vi "Do.vi"(8 "error in (no error)":errorcluster, 10 "Actor in":refnum<class "Actor.lvclass">, 11 "lfieldpanel_acquire_single_frame Msg":refnum<class "lfieldpanel_acquire_single_frame Msg.lvclass">) -> (0 "error out":errorcluster, 2 "Actor out":refnum<class "Actor.lvclass">)   [LabVIEW 2015, in "lfieldpanel_acquire_single_frame Msg.lvclass"]
doc: "This VI delivers the message to the actor by calling the appropriate method(s) on the actor."
uses:
  lfieldpanel_acquire_single_frame Msg.lvclass
  <vilib>/ActorFramework/Actor/Actor.lvclass
  lightfield_panel/lightfield_panel.lvclass
  lfieldpanel_acquire_single_frame Msg.lvclass/lfieldpanel_acquire_single_frame Msg.ctl
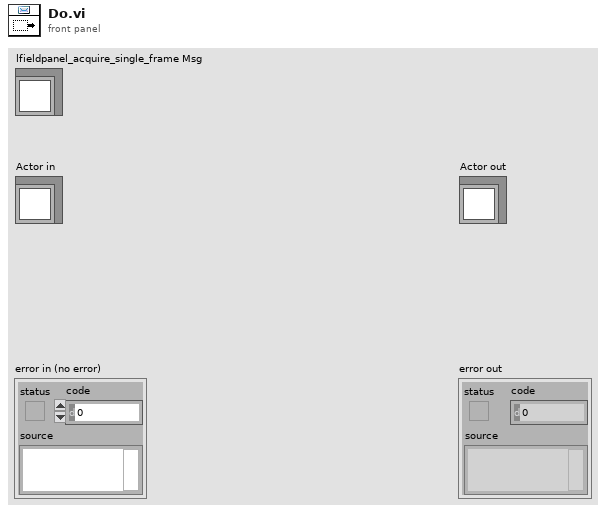
[diagram p1: front panel]
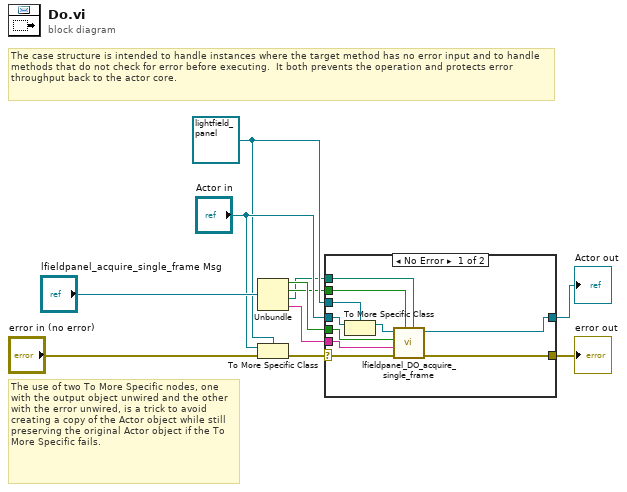
[diagram p0: block diagram]
diagram:
  w5 = refnum<class "lightfield_panel.lvclass"> refnum ("Actor in")
  # "The use of two To More Specific nodes, one with the output object unwired and the other with the error unwired, is a trick to avoid creating a copy of the Actor object while still preserving the original Actor object if the To More Specific fails."
  # "The case structure is intended to handle instances where the target method has no error input and to handle methods that do not check for error before executing.  It both prevents the operation and protects error throughput back to the actor core."
  n1 = Unbundle("lfieldpanel_acquire_single_frame Msg") -> (w4:bool, w3:bool, w2:path, w1:string)
  n2 = To More Specific Class(target class=w5, reference="Actor in", error in="error in (no error)") -> (error out=w9:errorcluster)  [unwired: 1 out]
  n3 = case shown="No Error" w9 {
    selector: w9 -> [w19 w23]
    tunnel: [w21 w23] -> w8
    tunnel: [w20 w22] -> w7
    tunnel: "Actor in" -> [w18 w22]
    tunnel: w5 -> [w17 _]
    tunnel: w4 -> [w15 _]
    tunnel: w3 -> [w14 _]
    tunnel: w2 -> [w13 _]
    tunnel: w1 -> [w12 _]
    frame No Error {
      n4 = To More Specific Class(target class=w17, reference=w18) -> (specific class reference=w16:refnum<class "lightfield_panel.lvclass">)  [unwired: 1 in, 1 out]
      n5 = call "lfieldpanel_DO_acquire_single_frame.vi"("savepath"=w13, "Log data"=w14, "error in (no error)"=w19, "notes"=w12, "Integrate_sensor"=w15, "lightfield_panel in"=w16) -> ("error out"=w21:errorcluster, "lightfield_panel out"=w20:refnum<class "lightfield_panel.lvclass">)  [unwired: 4 in]
    }
    frame Error {
      # "If type check fails, pass the original object out again."
    }
  }
  "error out" <- w8
  "Actor out" <- w7
